vi "Create instrument driver 'Read me' HTML file.vi"() -> ()   [LabVIEW 2012]
doc: "VI Description text"
uses:
  <vilib>/Platform/browser.llb/Open URL in Default Browser (path).vi
panel:
  in  "error in (no error)":errorcluster
  out "error out":errorcluster
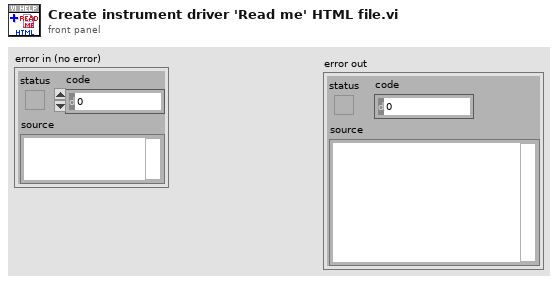
[diagram p1: front panel]
types:
  T1 = enum32{"Invalid", "Standard", "Closed", "Hidden", "Minimized", "Maximized"}
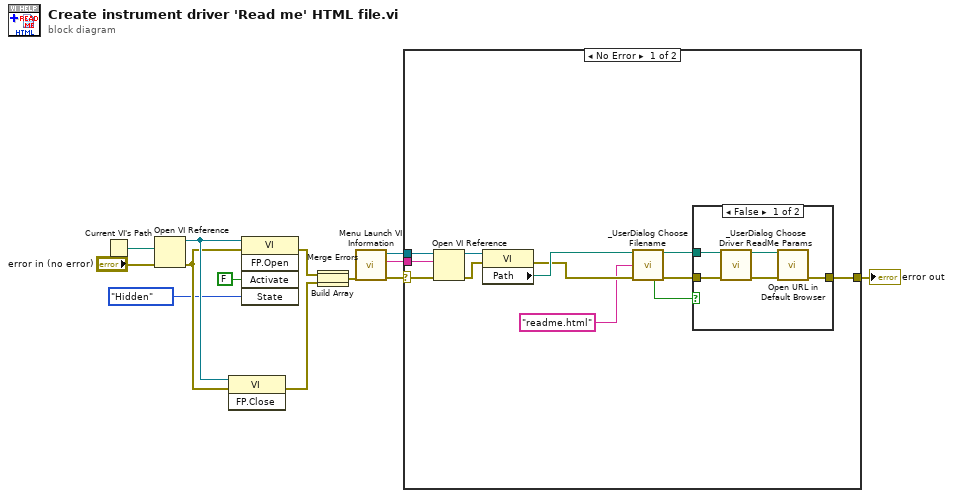
[diagram p0: block diagram]
diagram:
  n1 = Current VI's Path() -> (path=w7:path)
  n2 = Open VI Reference(vi path=w7, error in (no error)="error in (no error)") -> (vi reference=w5:refnum<vi>, error out=w4:errorcluster)  [unwired: 4 in]
  n3 = invoke class="VI" method="FP.Close"(reference=w5, error in=w4) -> (error out=w10:errorcluster)  [unwired: 1 in, 2 out]
  n4 = invoke class="VI" method="FP.Open"(reference=w5, error in=w4, "Activate"=FALSE ("Activate?"), "State"=T1."Hidden") -> (error out=w3:errorcluster)  [unwired: 1 in, 4 out]
  n5 = Build Array(w3, w10) -> (w6:errorcluster[])
  n6 = Merge Errors(w6) -> (w9:errorcluster)
  n7 = call <vilib>:"Menu Launch VI Information.vi"("error in (no error)"=w9) -> ("error out"=w12:errorcluster, "Menu Launch:VI"=w13:string, "Menu Launch:App"=w14:refnum<vi>)  [unwired: 8 in]
  n8 = case shown="No Error" w12 {
    selector: w12 -> [w24 w33]
    tunnel: [w19 w33] -> w11
    tunnel: w14 -> [w26 _]
    tunnel: w13 -> [w25 _]
    frame No Error {
      n9 = Open VI Reference(application reference (local)=w26, vi path=w25, error in (no error)=w24) -> (vi reference=w23:refnum<vi>, error out=w22:errorcluster)  [unwired: 3 in]
      n10 = property class="VI"(reference=w23, error in=w22) -> (error out=w20:errorcluster, "Path"=w21:path)  [unwired: 1 out]
      n11 = call "_UserDialog Choose Filename.vi"("VI Default Path"=w21, "Default file name"="readme.html" ("string"), "error in (no error)"=w20) -> ("HTML File Path"=w18:path, "Cancelled by User?"=w16:bool, "error out"=w17:errorcluster)  [unwired: 8 in, 2 out]
      n12 = case shown="False" w16 {
        tunnel: [w28 w32] -> w19
        tunnel: w18 -> [w31 _]
        tunnel: w17 -> [w30 w32]
        frame False {
          n13 = call "_UserDialog Choose Driver ReadMe Params.vi"("VI Default Path"=w31, "error in (no error)"=w30) -> ("HTML File Path"=w27:path, "error out"=w29:errorcluster)  [unwired: 11 in, 1 out]
          n14 = call-poly <vilib>:"Open URL in Default Browser.vi"("error in (no error)"=w29, "path"=w27) -> ("error out"=w28:errorcluster)  [unwired: 4 in, 1 out]
        }
        frame True {
        }
      }
    }
    frame Error {
    }
  }
  "error out" <- w11
